vi "Scale.vi"(0 "VISA IN":refnum<visa-resource-name>, 1 "Trace":i32=1, 2 "Scale Per Division":i32=1, 3 "Ref Level":i32=1, 4 "Ref Position":i32, 5 "error in":errorcluster, 7 "Window":i32=1) -> (14 "VISA Out":refnum<visa-resource-name>, 19 "error out":errorcluster)   [LabVIEW 2018, in "PNA-X.lvlib"]
uses:
  PNA-X.lvlib
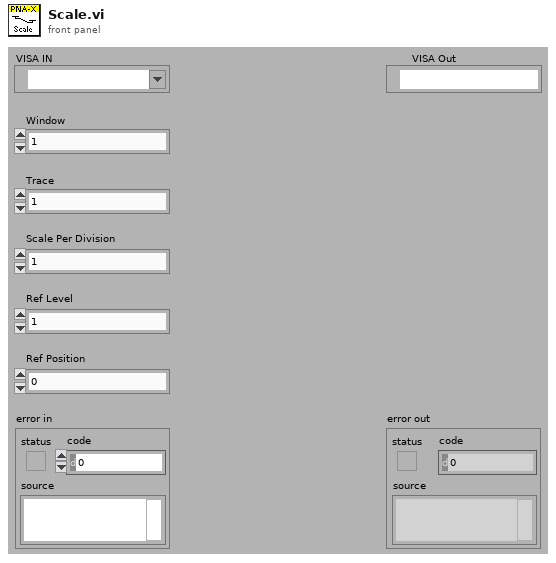
[diagram p1: front panel]
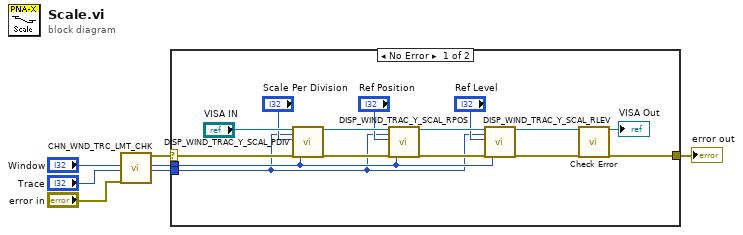
[diagram p0: block diagram]
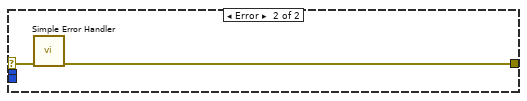
[diagram p2: hidden frame]
diagram:
  n1 = call "CHN_WND_TRC_LMT_CHK.vi"("Window"="Window", "Trace"="Trace", "error in"="error in") -> ("error out"=w4:errorcluster, "Window"=w2:i32, "Trace"=w1:i32)  [unwired: 12 in, 2 out]
  n2 = case shown="No Error" w4 {
    selector: w4 -> [w20 w24]
    tunnel: [w22 w23] -> w5
    tunnel: w2 -> [w16 _]
    tunnel: w1 -> [w8 _]
    frame No Error {
      n3 = call "DISP_WIND_TRAC_Y_SCAL_PDIV.vi"("VISA IN"="VISA IN", "Trace"=w8, "Division"="Scale Per Division", "error in"=w20, "Window"=w16) -> ("VISA Out"=w14:refnum<visa-resource-name>, "error out"=w19:errorcluster)  [unwired: 13 in]
      n4 = call "DISP_WIND_TRAC_Y_SCAL_RPOS.vi"("VISA IN"=w14, "Trace"=w8, "Position"="Ref Position", "error in"=w19, "Window"=w16) -> ("VISA Out"=w13:refnum<visa-resource-name>, "error out"=w18:errorcluster)  [unwired: 13 in]
      n5 = call "DISP_WIND_TRAC_Y_SCAL_RLEV.vi"("VISA IN"=w13, "Trace"=w8, "Ref Level"="Ref Level", "error in"=w18, "Window"=w16) -> ("VISA Out"=w12:refnum<visa-resource-name>, "error out"=w17:errorcluster)  [unwired: 13 in]
      n6 = call "Check Error.vi"("VISA Resource Name"=w12, "error in (no error)"=w17) -> ("dup VISA session"=→"VISA Out":refnum<visa-resource-name>, "error out"=w22:errorcluster)  [unwired: 16 in]
    }
    frame Error {
      n7 = call <vilib>:"Simple Error Handler.vi"("error in (no error)"=w24) -> ("error out"=w23:errorcluster)  [unwired: 4 in, 4 out]
    }
  }
  "error out" <- w5
